vi "lissajous_3d.vi"() -> ()   [LabVIEW 2021]
uses:
  <vilib>/Math Plots/3D Math Plots/3D Comet/3D Comet XCtrl/3D Comet.xctl
  <vilib>/Math Plots/3D Math Plots/3D Comet/3D Comet Datatype/Public/Plot Helper (Vector).vi
  <vilib>/Math Plots/3D Math Plots/3D Comet/3D Comet Datatype/3D Comet Datatype.lvclass
panel:
  out "3D Comet":refnum<class "3D Plot Datatype.lvclass">[](xcontrol)
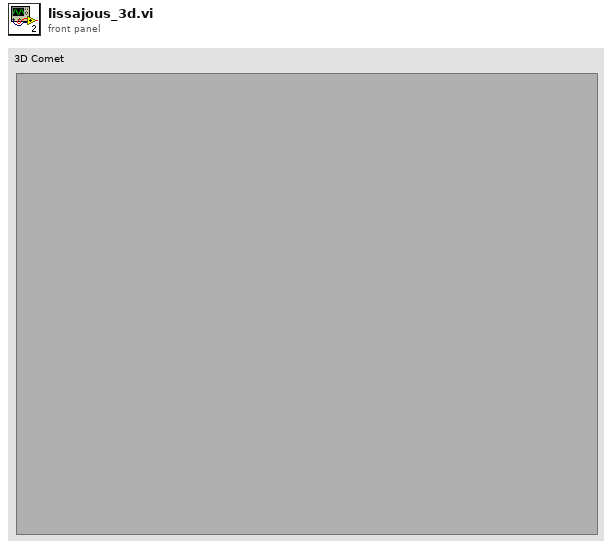
[diagram p1: front panel]
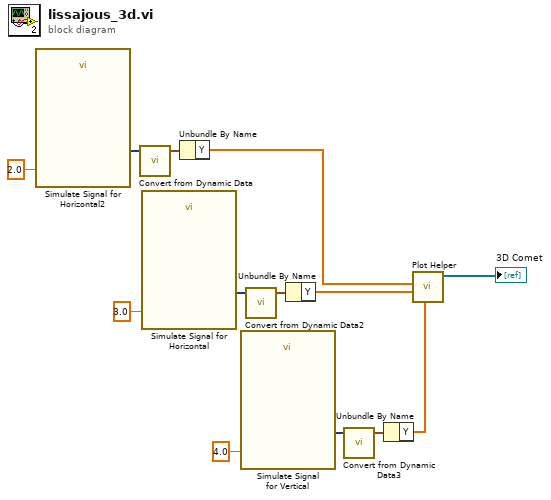
[diagram p0: block diagram]
diagram:
  n1 = call "Simulate Signal for Horizontal2"("Frequency"=2.0) -> ("Sine"=w10:dynamicdata)  [unwired: 5 in, 9 out]
  n2 = call "Convert from Dynamic Data"("Dynamic Data Type"=w10) -> ("Waveform"=w9:waveform(dbl))  [unwired: 3 in]
  n3 = call "Simulate Signal for Horizontal"("Frequency"=3.0) -> ("Sine"=w6:dynamicdata)  [unwired: 5 in, 9 out]
  n4 = Unbundle By Name(w9) -> ("Y"=w3:dbl[])
  n5 = call "Simulate Signal\nfor Vertical"("Frequency"=4.0) -> ("Sine"=w5:dynamicdata)  [unwired: 5 in, 9 out]
  n6 = call "Convert from Dynamic Data2"("Dynamic Data Type"=w6) -> ("Waveform"=w8:waveform(dbl))  [unwired: 3 in]
  n7 = Unbundle By Name(w8) -> ("Y"=w2:dbl[])
  n8 = call "Convert from Dynamic Data3"("Dynamic Data Type"=w5) -> ("Waveform"=w7:waveform(dbl))  [unwired: 3 in]
  n9 = Unbundle By Name(w7) -> ("Y"=w1:dbl[])
  n10 = call-poly <vilib>:"Plot Helper.vi"("z vector"=w1, "y vector"=w2, "x vector"=w3) -> ("3D Plot lvclass Array out"=→"3D Comet":refnum<class "3D Plot Datatype.lvclass">[])  [unwired: 3 in, 5 out]
